vi "String to I32.vi"(8 "error in (no error)":errorcluster, 11 "String to Convert":string) -> (0 "error out":errorcluster, 3 "I32 Value":i32 format="%.0g")   [LabVIEW 2023, in "HAF.lvlib"]
doc: "Conerts a passed String into a signed 32-bit integer."
uses:
  HAF.lvlib
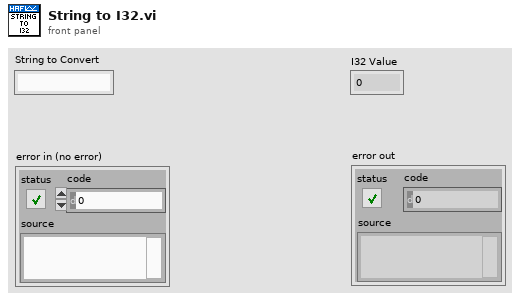
[diagram p1: front panel]
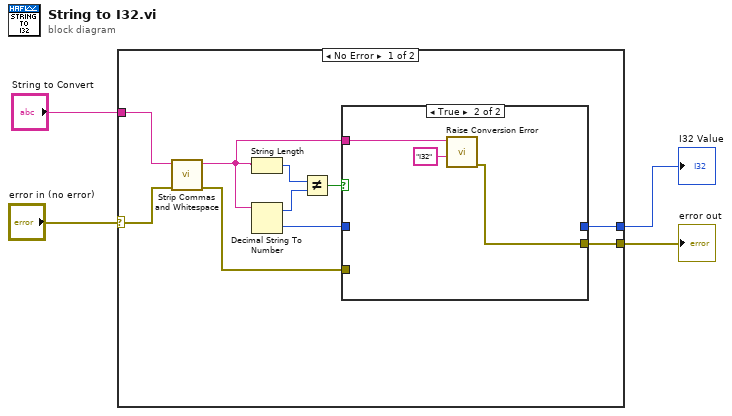
[diagram p0: block diagram]
diagram:
  n1 = case shown="No Error" "error in (no error)" {
    selector: "error in (no error)" -> [w13 w20]
    tunnel: "String to Convert" -> [w14 _]
    tunnel: [w7 w20] -> w2
    tunnel: [w5 _] -> w1
    frame No Error {
      n2 = call "Strip Commas and Whitespace.vi"("error in (no error)"=w13, "String to Strip"=w14) -> ("error out"=w6:errorcluster, "Clean String"=w9:string)  [unwired: 8 in]
      n3 = String Length(string=w9) -> (length=w12:i32)
      n4 = Decimal String To Number(string=w9) -> (offset past number=w11:i32, number=w8:i32)  [unwired: 2 in]
      n5 = Not Equal?(x=w12, y=w11) -> (x != y?=w10:bool)
      n6 = case shown="True" w10 {
        tunnel: w9 -> [_ w19]
        tunnel: w8 -> [w15 _]
        tunnel: [w16 w17] -> w7
        tunnel: w6 -> [w16 _]
        tunnel: [w15 _] -> w5
        frame False {
        }
        frame True {
          n7 = call "Raise Conversion Error.vi"("Data Type Attempted"="I32", "String in Error"=w19) -> ("error out"=w17:errorcluster)  [unwired: 9 in]
        }
      }
    }
    frame Error {
    }
  }
  "I32 Value" <- w1
  "error out" <- w2
